vi "cmd_note.vi"(8 "error in (no error)":errorcluster, 11 "JSON":string) -> (0 "error out":errorcluster)   [LabVIEW 2021]
doc: "Call note command\n\n This is just for taking a note in the log file\n\n :param note: Note"
panel:
  in  "args":cluster{"note":string}
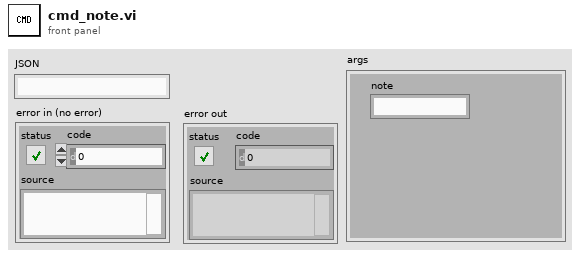
[diagram p1: front panel]
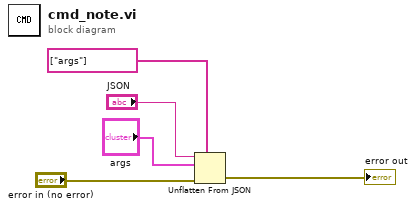
[diagram p0: block diagram]
diagram:
  n1 = Unflatten From JSON(path=string[] ["args"], JSON string="JSON", type and defaults="args", error in (no error)="error in (no error)") -> (error out=→"error out":errorcluster)  [unwired: 3 in, 1 out]
